vi "Close.vi"(8 "error in (no error)":errorcluster, 11 "Carya Config (Buffer) in":refnum<class "CConfig Buffer Type.lvclass">) -> (0 "error out":errorcluster)   [LabVIEW 2013, in "CConfig Buffer Type.lvclass"]
doc: "Copyright 2018, Carya Automatisering, Wiebe Walstra."
uses:
  CConfig Buffer Type.lvclass
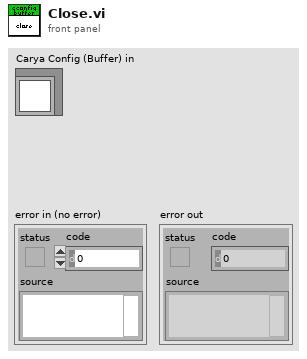
[diagram p1: front panel]
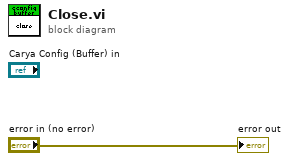
[diagram p0: block diagram]
diagram:
  "error out" <- "error in (no error)"
